vi "LVFunction_Imop_Compute_ZonalWavefront.vi"(0 "HasoData.lvclass":refnum<class "HasoData.lvclass">, 5 "ComputePhaseSet.lvclass":refnum<class "ComputePhaseSet.lvclass">, 7 "Phase":refnum<class "Phase.lvclass">, 11 "error constant":errorcluster) -> (4 "HasoData.lvclass (dup)":refnum<class "HasoData.lvclass">, 6 "ComputePhaseSet.lvclass 2":refnum<class "ComputePhaseSet.lvclass">, 8 "Phase":refnum<class "Phase.lvclass">, 15 "error out":errorcluster)   [LabVIEW 2020]
doc: "Compute phase from processed slopes of the input HasoData.\n\nFilter some aberrations of reconstructed phase, depending on the filter given in zonal phase reconstruction parameters providing by ComputePhaseSet.\n\n<B>ComputePhaseSetIn</B> : ComputePhaseSet object.\n<B>ComputePhaseSetOut</B> : ComputePhaseSet object.\n<B>HasoData</B> : HasoData object.\n<B>Phase</B> : phase object. Phase unit is um. Phase sampling steps unit is um."
uses:
  HasoData.lvclass
  ComputePhaseSet.lvclass
  Phase.lvclass
  LVClasse_Phase Read SurfaceFloatWithPupil.vi
  LVClass_ComputePhaseSet Read ComputePhaseSet.vi
  LVClass_HasoData Read HasoData - property.vi
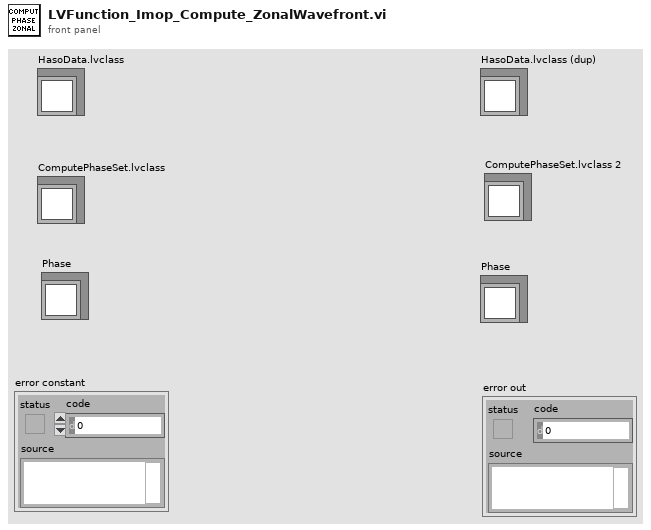
[diagram p1: front panel]
types:
  T1 = typedef "ClassID.ctl" = i64
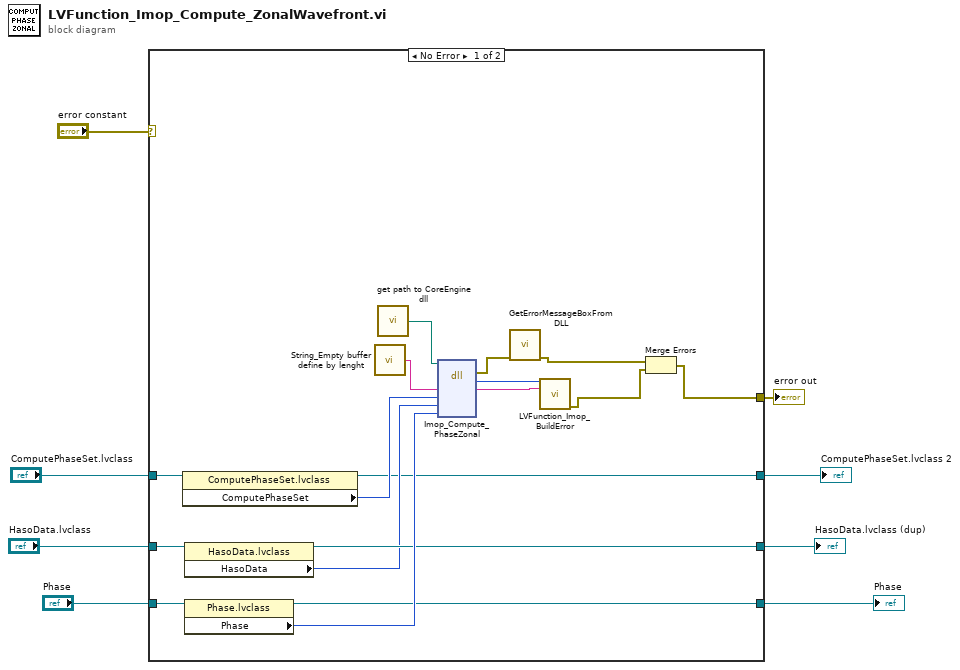
[diagram p0: block diagram]
diagram:
  n1 = case shown="No Error" "error constant" {
    selector: "error constant" -> [_ w29]
    tunnel: "HasoData.lvclass" -> [w20 w27]
    tunnel: "ComputePhaseSet.lvclass" -> [w19 w26]
    tunnel: [w14 w29] -> w6
    tunnel: "Phase" -> [w18 w28]
    tunnel: [w13 w28] -> w3
    tunnel: [w11 w27] -> w2
    tunnel: [w9 w26] -> w1
    frame No Error {
      n2 = property class="ComputePhaseSet.lvclass"(reference=w19) -> (reference out=w9:refnum<class "ComputePhaseSet.lvclass">, "ComputePhaseSet"=w12:T1)  [unwired: 1 in, 1 out]
      n3 = property class="HasoData.lvclass"(reference=w20) -> (reference out=w11:refnum<class "HasoData.lvclass">, "HasoData"=w10:T1)  [unwired: 1 in, 1 out]
      n4 = property class="Phase.lvclass"(reference=w18) -> (reference out=w13:refnum<class "Phase.lvclass">, "Phase"=w17:T1)  [unwired: 1 in, 1 out]
      n5 = call "String_Empty buffer define by lenght.vi"() -> ("Empty buffer"=w23:string)  [unwired: 1 in]
      n6 = call "get path to CoreEngine dll.vi"() -> ("path to wavekit library"=w22:path)  [unwired: 14 in, 1 out]
      n7 = dll-call lib="D:/FLE/0.Code/CoreEngine4_Suite/LV2011_interface/DLLs/c_interface_vc100.dll" fn="Imop_Compute_PhaseZonal"(path in=w22, "message"=w23, "ComputePhaseSet"=w12, "HasoData"=w10, "phase"=w17) -> (error out=w21:errorcluster, "return type"=w25:i32, "message"=w24:string)  [unwired: 5 in, 1 out]
      n8 = call "GetErrorMessageBoxFromDLL.vi"("error IN"=w21) -> ("error OUT"=w16:errorcluster)  [unwired: 10 in]
      n9 = call "LVFunction_Imop_BuildError.vi"("code"=w25, "String to Prepend to source (\"\")"=w24) -> ("error out"=w15:errorcluster)  [unwired: 13 in]
      n10 = Merge Errors(w16, w15) -> (w14:errorcluster)
    }
    frame Error {
    }
  }
  "error out" <- w6
  "Phase" <- w3
  "HasoData.lvclass (dup)" <- w2
  "ComputePhaseSet.lvclass 2" <- w1
